vi "Main.vi"() -> ()   [LabVIEW 2013] (continued)
      n78 = control-ref of="Item Details"() -> (w112:refnum<vi>)
      n79 = control-ref of="WPS Details Setup"() -> (w111:refnum<vi>)
      n80 = control-ref of="Info. (Execute Page)"() -> (w96:refnum<vi>)
      n81 = control-ref of="Results Output"() -> (w72:refnum<vi>)
      n82 = control-ref of="Furnace Details"() -> (w98:refnum<vi>)
      n83 = control-ref of="Extra WPS"() -> (w110:refnum<vi>)
      n84 = control-ref of="Extra Rev"() -> (w109:refnum<vi>)
      n85 = control-ref of="Notes"() -> (w107:refnum<vi>)
      n86 = Initialize Array("", w121) -> (w242:string[])
      n87 = control-ref of="This Application"() -> (w187:refnum<vi>)
      n88 = Initialize Array("", w228) -> (w231:string[])
      n89 = Initialize Array("", w134) -> (w240:string[])
      n90 = property on="Tab Body" class="TabCtl (strict)" props=["Pages"]() -> ()  [unwired: 2 in, 3 out]
      n91 = property on="Tab Setup" class="TabCtl (strict)" props=["Pages"]() -> ()  [unwired: 2 in, 3 out]
      n92 = property on="Master Data Tab" class="TabCtl (strict)" props=["Pages"]() -> ()  [unwired: 2 in, 3 out]
      n93 = property class="App"(reference=w187) -> (error out=w142:errorcluster, "App.Dir"=w149:path, "App.Name"=w148:string)  [unwired: 1 in, 1 out]
      "Application:Name" <- w148
      "LabVIEW Directory Path" <- w149
      n94 = Build Array(w242) -> (w243:string[][])
      n95 = Build Array(w231) -> (w230:string[][])
      n96 = Build Array(w240) -> (w133:string[][])
      n97 = control-ref of="Equipment Details"() -> (w157:refnum<vi>)
      n98 = control-ref of="FTP File List"() -> (w126:refnum<vi>)
      n99 = control-ref of="Report List"() -> (w153:refnum<vi>)
      n100 = control-ref of="Part Details"() -> (w233:refnum<vi>)
      n101 = property on="MCListBox FHS Setup" class="MCListbox (strict)"("ItemNames"=w230, "NumCols"=w228, "ColHdrString"=w199) -> ()  [unwired: 2 in, 2 out]
      n102 = property on="MCListBox FHS Master Data" class="MCListbox (strict)"("ItemNames"=w243, "NumCols"=w121, "ColHdrString"=w199) -> ()  [unwired: 2 in, 2 out]
      n103 = property on="MCListBox AWPS" class="MCListbox (strict)"("ItemNames"=w133, "NumCols"=w134) -> ()  [unwired: 2 in, 2 out]
      n104 = Bundle By Name(cluster=T23 {"Item Details"=refnum, "WPS Details"=refnum, "WPS (Extra)"=refnum, "Rev (Extra) "=refnum, "FHS MCListbox"=refnum, "Additional WPS/Ref MCListBox"=refnum, "Notes"=refnum, "Part Details (MClistBox)"=refnum, "Result Output"=refnum} ("Refnums"), "Item Details"=w112, "WPS Details"=w111, "WPS (Extra)"=w110, "Rev (Extra)"=w109, "FHS MCListbox"=w114, "Additional WPS/Ref MCListBox"=w108, "Notes"=w107, "Part Details (MClistBox)"=w106, "Result Output"=w72) -> (→"DB Refnums":T23)
      n105 = Bundle By Name(cluster=T24 {"Furnace Details"=refnum, "CompactRIO Module Details"=refnum, "Info. (Execute Tab)"=refnum} ("DB Refnums II"), "Furnace Details"=w98, "CompactRIO Module Details"=w97, "Info. (Execute Tab)"=w96) -> (→"DB Refnums II":T24)
      n106 = control-ref of="MCListBox FHS Setup"() -> (w118:refnum<vi>)
      n107 = control-ref of="MCListBox FHS Master Data"() -> (w120:refnum<vi>)
      n108 = control-ref of="MCListBox AWPS"() -> (w179:refnum<vi>)
      n109 = property on="Material Copy" class="Bool"("DisabledEnum"=T30."Disabled and Grayed Out" ("Disabled")) -> ()  [unwired: 2 in, 2 out]
      n110 = property on="Material Paste" class="Bool"("DisabledEnum"=T30."Disabled and Grayed Out" ("Disabled")) -> ()  [unwired: 2 in, 2 out]
      n111 = Build Path(base path=w149, name or relative path=w148) -> (appended path=w147:path)
      n112 = Path To String(path=w147) -> (string=w146:string)
      n113 = invoke class="FileVersionInfo" method="GetVersionInfo"(error in=w142, "fileName"=w146) -> (reference out=w143:refnum<k24>, error out=w141:errorcluster, "GetVersionInfo"=w145:refnum<k24>)  [unwired: 2 in, 1 out]
      n114 = property class="MCListbox (strict)"(reference=w233, "ColHdrString"=w232, "NumRows"=w135, "NumCols"=u32 19 ("Number of Rows")) -> (reference out=w136:refnum<vi>)  [unwired: 1 in, 1 out]
      n115 = for {
        N: w135 -> [_]
        tunnel: w136 -> [w302]
        i -> [w301]
        n116 = for {
          N: 6 -> [_]
          tunnel: w302 -> [w309]
          tunnel: w301 -> [w306]
          tunnel: 13 -> [w305]
          i -> [w304]
          n117 = Add(x=w305, y=w304) -> (x+y=w303:i32)
          n118 = Bundle(w306, w303) -> (w307:cluster{i32, i32})  [unwired: 1 in]
          n119 = property class="MCListbox (strict)"(reference=w309, "ActiveCell"=w307, "Justify"=enum16{"Left", "Center", "Right"}."Center" ("Active Cell:Cell Justification")) -> ()  [unwired: 1 in, 2 out]
        }
      }
      n120 = property class="MCListbox (strict)"(reference=w157, "ColHdrString"=w154, "NumRows"=u32 4 ("Number of Rows"), "NumCols"=u32 5 ("Number of Rows")) -> (reference out=w156:refnum<vi>)  [unwired: 1 in, 1 out]
      n121 = property class="MCListbox (strict)"(reference=w153, "ColHdrString"=w150, "NumRows"=u32 5 ("Number of Rows"), "NumCols"=u32 7 ("Number of Rows")) -> (reference out=w152:refnum<vi>)  [unwired: 1 in, 1 out]
      n122 = property class="MCListbox (strict)"(reference=w126, "ColHdrString"=string[] ["Date and Time", "Transaction No."] ("Column Header Strings[]"), "NumRows"=u32 5 ("Number of Rows"), "NumCols"=u32 2 ("Number of Rows")) -> (reference out=w123:refnum<vi>)  [unwired: 1 in, 1 out]
      n123 = property on="Property Node" class="MCListbox (strict)"(reference=w120, "NumRows"=8 ("Multicolumn Listbox"), "TopLeft"=w173) -> ()  [unwired: 1 in, 2 out]
      n124 = property on="Property Node" class="MCListbox (strict)"(reference=w118, "NumRows"=8 ("Multicolumn Listbox"), "TopLeft"=w173) -> ()  [unwired: 1 in, 2 out]
      n125 = local write "Close"(FALSE ("Quit")) -> ()
      n126 = Build Array(w118, w120, w179) -> (w190:refnum<vi>[])
      "MCListBox Ref" <- w190
      n127 = property on="Part Details Add" class="Bool (strict)"("BoolText.Text"="Add" ("Boolean Text.Text"), "DisabledEnum"=T30."Enabled" ("Disabled")) -> ()  [unwired: 2 in, 2 out]
      n128 = property class="FileVersionInfo"(reference=w145, error in=w141) -> (reference out=w144:refnum<k24>, error out=w140:errorcluster, "FileVersion"=w137:string)
      n129 = for {
        tunnel: w190 -> [w362] mode=indexing
        tunnel: "CellBG Unused Cells" -> [w365]
        tunnel: "CellBG ColHdrs" -> [w364]
        tunnel: "CellBG New Cells" -> [_]
        n130 = property on="Property Node" class="MCListbox (strict)"(reference=w362, "RowHdrs[]"=string[] ["-1,-1", "", "0,0", "-1,-1", "7"]) -> (reference out=w361:refnum<vi>)  [unwired: 1 in, 1 out]
        n131 = property on="Property Node" class="MCListbox (strict)"(reference=w361, "ActiveCell"=T33 {"Row"=-2, "Column"=-2}, "CellBG"=w365, "ActiveCell"=T33 {"Row"=-1, "Column"=-2}, "CellBG"=w364, "Value"=-1 ("Multicolumn Listbox")) -> ()  [unwired: 1 in, 2 out]
      }
      n132 = Concatenate Strings("ver. ", w137) -> (w51:string)
      "File Version" <- w51
      n133 = flat-sequence "RSS Copyright" {
        frame #0 {
          # "Copyright (c) 2014, Reinehold Systems Solutions Pte Ltd. All Rights Reserved.\n\nThis application code (VI) is confidential and/or proprietary and is intended for the express use of the copyright owner and/or IP owner. This code is delivered as part of the Stress Relief Recording System. Any unauthorized re-use of this code outside of the Stress Relief Recording System is prohibited and punishable by law."
        }
      }
      n134 = flat-sequence "Report TAB" {
        frame #0 {
        }
      }
      n135 = Close Reference(reference=w144, error in (no error)=w140) -> (error out=w139:errorcluster)
      n136 = call "Get INFO from ini FILE - SRTRS.vi"("ini Name"="SRTRS.ini") -> ("Settings"=w56:T37, "Equipment Details (MCListBox)"=w214:string[][], "Furnace Details"=→"Furnace Details":T6, "SRTRS Connection Information"=w92:T38, "CMS Connection Information"=w80:T38, "AMS Connection Information"=w49:T38, "MessageQ"=w185:string, "Settings Boolean"=w48:T39, "Error Out"=w77:errorcluster)  [unwired: 5 in, 1 out]
      "ini File Error" <- w77
      n137 = Unbundle By Name(w56) -> ("cRIO IP"=w196:string, "Host COM Port"=w57:string, "Temperature Units"=w84:string, "cRIO Folder"=→"cRIO Folder":string, "cRIO Data Retention"=w177:string, "cRIO Time Sync Schedule"=w63:string, "cRIO Time Sync Tolerance"=w64:string, "Furnace Number"=→"Furnace Number":string, "Software Solution Name"=→"ApplicationName":string, "LogoFile"=w90:string, "Channel to Probe Mapping"=w211:string, "Running Number"=w213:string, "Permitted Temperature Difference"=w201:string, "Host Sampling Interval"=w189:string, "Latest stp File"=w131:string, "Log Off Timer"=w91:string, "Raw Data File"=→"Raw Data File":string, "SRTRS4070 Host Folder"=w36:string, "SRTRS4070 Folder"=→"SRTRS4070 Folder (Server Folder)":string, "Layout Details"=w34:string, "Date Format"=w26:string)  [unwired: 1 out]
      "cRIO IP" <- w196
      "Host COM Port" <- w57
      "SRTRS4070 Host Folder" <- w36
      n138 = Close Reference(reference=w143, error in (no error)=w139) -> ()  [unwired: 1 out]
      n139 = Build Array(w136, w156, w152, w123) -> (w244:refnum<vi>[])
      n140 = local read "CellBG Unused Cells"() -> (w234:u32)
      n141 = Concatenate Strings("{Initialization} SRTRS Initialize OK." ("string"), w185, " " ("string"), w181) -> (w28:string)
      n142 = Unbundle By Name "Settings Boolean"(w48) -> ("Create EXCEL"=w205:bool, "Create PDF"=w204:bool, "Use Host COM Port"=w195:bool, "Show LabVIEW Error"=→"Show LabVIEW Error":bool, "Show Debug Tab"=w39:bool, "Show Scrollbars"=w163:bool, "Stop On Final Target Temperature"=w129:bool, "Update English Captions"=w40:bool)
      "Show Debug TAB" <- w39
      "Show Scrollbars" <- w163
      "Update English Captions" <- w40
      n143 = Select(t=T31."Always On" ("Vertical Scrollbar Visibility"), s=w163, f=T31."Off While Running" ("Vertical Scrollbar Visibility")) -> (s? t:f=w160:T31)
      n144 = property class="Pane"(reference=w164, "HorizScrollbarVisibility"=w160, "VertScrollbarVisibility"=w160) -> ()  [unwired: 1 in, 2 out]
      n145 = Unbundle By Name "Settings Boolean"(w48) -> ("Simulate cRIO"=w47:bool, "Simulate ET3500"=w46:bool, "Simulate No DB"=w44:bool, "Lite Version"=w45:bool)
      "Lite Version" <- w45
      n146 = case shown="True" "DB - Logon" {
        frame False {
        }
        frame True {
          n147 = property on="Close" class="Bool (strict)"("BoolText.Text"="Log off" ("Label.Text")) -> (error out=w276:errorcluster)  [unwired: 2 in, 1 out]
          n148 = property on="Close" class="Bool (strict)"(error in=w276, "Val(Sgnl)"=TRUE ("Value (Signaling)")) -> ()  [unwired: 1 in, 2 out]
        }
      }
      n149 = for {
        tunnel: w244 -> [w371] mode=indexing
        tunnel: w234 -> [w370]
        tunnel: string[][] [] ("Item Names") -> [w369]
        w372 = T33 {"Row"=-1, "Column"=-2}  # All ColHdrs
        w373 = T33 {"Row"=-2, "Column"=-2}  # All Rows & Columns (Including Headers)
        n150 = property on="Property Node" class="MCListbox (strict)"(reference=w371, "ActiveCell"=w373, "CellBG"=w370, "ActiveCell"=w372, "CellBG"=u32 12105912, "ItemNames"=w369) -> ()  [unwired: 1 in, 2 out]
      }
      n151 = Reverse String(1:w51) -> (0:w52:string)
      n152 = local write "Date Format (UserDefined)"(w26) -> ()
      n153 = Match Pattern(string=w52, regular expression="\\." ("search string")) -> (after substring=w54:string)  [unwired: 1 in, 3 out]
      n154 = flat-sequence "MasterData TAB (xx Controls)" {
        frame #0 {
          n155 = property on="SAPMaterial Description (Long) Master Data Tab" class="Bool"("DisabledEnum"=T30."Disabled and Grayed Out" ("Disabled")) -> ()  [unwired: 2 in, 2 out]
          n156 = property on="Master Data Material Description" class="Str"("Text.BGColor"=u32 16777215, "DisabledEnum"=T30."Enabled" ("Disabled")) -> ()  [unwired: 2 in, 2 out]
          n157 = property on="Material Save" class="Bool"("DisabledEnum"=T30."Disabled and Grayed Out" ("Disabled")) -> ()  [unwired: 2 in, 2 out]
        }
      }
      n158 = Search and Replace String(input string="ni.var.psp://cRIO IP/RT Library" ("String"), search string="cRIO IP" ("String"), replace string=w196) -> (result string=→"cRIO shared variable RT Library":string)  [unwired: 5 in, 3 out]
      n159 = Search and Replace String(input string="visa://cRIO IP/ASRL1::INSTR" ("String"), search string="cRIO IP" ("String"), replace string=w196) -> (result string=w194:string)  [unwired: 5 in, 3 out]
      "cRIO COM Port" <- w194
      n160 = Reverse String(1:w54) -> (0:→"Plant and Furnace Name" →"Plant and Furnace Name (B4 Logon)":string)
      n161 = local write "Use Host COM Port"(w195) -> ()
      n162 = local write "Report.Create.Excel"(w205) -> ()
      n163 = local write "Report.Create.PDF"(w204) -> ()
      n164 = global write "Global SRTRS.vi" "SRTRS Connection Information"(w92) -> ()
      n165 = global write "Global SRTRS.vi" "CMS Connection Information"(w80) -> ()
      n166 = global write "Global SRTRS.vi" "AMS Connection Information"(w49) -> ()
      n167 = property on="Equipment Details" class="MCListbox (strict)"("ItemNames"=w214) -> ()  [unwired: 2 in, 2 out]
      n168 = global write "Global SRTRS.vi" "Update English Captions"(w40) -> ()
      n169 = Decimal String To Number(string=w177) -> (number=→"cRIO Data Retention":i32)  [unwired: 2 in, 1 out]
      n170 = Decimal String To Number(string=w64) -> (number=→"cRIO Time Sync Tolerance":i32)  [unwired: 2 in, 1 out]
      n171 = Match Pattern(string=w63, regular expression=":") -> (before substring=w61:string, after substring=w60:string)  [unwired: 1 in, 2 out]
      n172 = String To Path(string=w131) -> (path=→"Latest stp file":path)
      n173 = Bundle("Channel to Probe Mapping"=w211) -> (w172:cluster{"Channel to Probe Mapping":string})  [unwired: 1 in]
      n174 = Decimal String To Number(string=w213) -> (number=→"Running Number":i32)  [unwired: 2 in, 1 out]
      n175 = String To Path(string=w90) -> (path=w89:path)
      n176 = Fract/Exp String To Number(string=w201) -> (number=w200:dbl)  [unwired: 3 in, 1 out]
      n177 = Fract/Exp String To Number(string=w189) -> (number=→"Host Sampling Interval (s)":dbl)  [unwired: 3 in, 1 out]
      n178 = Decimal String To Number(string=w91) -> (number=→"Log Off Timer (s)":i32)  [unwired: 2 in, 1 out]
      n179 = Match Pattern(string=w34, regular expression="\t" ("search string/char (-)")) -> (before substring=→"Layout ID":string, after substring=w32:string)  [unwired: 1 in, 2 out]
      n180 = property on="Channel to Probe Mapping" class="Clust (strict)"("Value"=w172) -> ()  [unwired: 2 in, 2 out]
      n181 = Concatenate Strings(w61, w60) -> (w59:string)
      n182 = property on="Variant Allowed (Hold Temp)" class="DigNum (strict)"("Value"=w200) -> ()  [unwired: 2 in, 2 out]
      n183 = call <vilib>:"Read JPEG File.vi"("path to JPEG file"=w89) -> ("error out"=→"LogoName":errorcluster, "image data"=w88:T40)  [unwired: 8 in, 1 out]
      n184 = String To Path(string=w32) -> (path=→"Template File":path)
      n185 = case shown="True" "Edit WPS in Setup" {
        tunnel: w120 -> [w280 w282]
        tunnel: [w281 w284] -> w119
        tunnel: w118 -> [_ w283]
        frame False {
          # "Only Master FHS"
          n186 = Build Array(w280) -> (w281:refnum<vi>[])
        }
        frame True {
          # "Both FHS"
          n187 = Build Array(w283, w282) -> (w284:refnum<vi>[])
        }
      }
      n188 = Decimal String To Number(string=w59) -> (number=→"cRIO Time Sync Schedule":i32)  [unwired: 2 in, 1 out]
      n189 = call <vilib>:"Draw Flattened Pixmap.vi"("image data"=w88) -> ("new picture"=→"LogoName":picture)  [unwired: 8 in]
      n190 = case shown="True" w45 {
        tunnel: w47 -> [w296 _]
        tunnel: [w296 w298] -> w128
        tunnel: w46 -> [w295 _]
        tunnel: [w295 w298] -> w127
        frame False {
          # "Set Focus on Setup Tab"
          # "Full Version"
          n191 = property on="Tab Setup" class="TabCtl (strict)"("Value"=enum32{"Part Details", "Furnace Settings"}."Part Details" ("Tab Setup")) -> ()  [unwired: 2 in, 2 out]
        }
        frame True {
          w298 = TRUE ("Simulate cRIO")
          # "Simulate cRIO and ET3500"
          # "Lite Version"
        }
      }
      n192 = case shown="False" w44 {
        tunnel: [i32[] [0, 1, 2] i32[] [1]] -> w43
        tunnel: [TRUE FALSE] -> w42
        frame False {
          # "2 - Caption"
          # "DB Availiable"
        }
        frame True {
          # "Skip 0"
          # "Simulate No DB"
        }
      }
      "Settings Load Sequence" <- w43
      n193 = local write "Stop On Final Target Temperature"(w129) -> ()
      n194 = local write "From Search Button"(FALSE ("From Search Button")) -> ()
      n195 = for {
        tunnel: "CellBG New Cells" -> [w289]
        tunnel: w119 -> [w286] mode=indexing
        # "MClistbox FHS Setup \nis set to FALSE for\n\"Allowing Editing Cells\"\n/\"Editable Cells"
        # "Create WHITE\neditable cells"
        n196 = property on="Property Node" class="MCListbox (strict)"(reference=w286, "Allow Editing Cells"=TRUE) -> (reference out=w288:refnum<vi>, "NumCols"=w287:u32)  [unwired: 1 in, 1 out]
        n197 = for {
          N: w287 -> [_]
          tunnel: w289 -> [w291]
          tunnel: w288 -> [w290]
          i -> [w293]
          n198 = Bundle("Multicolumn Listbox"=0, w293) -> (w292:cluster{"Multicolumn Listbox":i32, i32})  [unwired: 1 in]
          n199 = property on="Property Node" class="MCListbox (strict)"(reference=w290, "ActiveCell"=w292, "CellBG"=w291) -> ()  [unwired: 1 in, 2 out]
        }
      }
      n200 = control-ref of="Logs_Host"() -> (w38:refnum<vi>)
      n201 = flat-sequence "Admin TAB (xx Controls)" {
        frame #0 {
        }
      }
      n202 = control-ref of="Master Data Temperature Units"() -> (w227:refnum<vi>)
      n203 = control-ref of="Key Values Temperature Units"() -> (w226:refnum<vi>)
      n204 = control-ref of="WPS Details Temperature Units"() -> (w225:refnum<vi>)
      n205 = control-ref of="Info. Temperature Units"() -> (w223:refnum<vi>)
      n206 = control-ref of="Info. Temperature Units 2"() -> (w222:refnum<vi>)
      n207 = control-ref of="FHS Ramp Rate Units"() -> (w209:refnum<vi>)
      n208 = control-ref of="FHS Target Temp Units"() -> (w208:refnum<vi>)
      n209 = control-ref of="MasterData FHS Ramp Rate Temp Units"() -> (w207:refnum<vi>)
      n210 = control-ref of="MasterData FHS Target Temp Units"() -> (w206:refnum<vi>)
      n211 = Select(t=w57, s=w195, f=w194) -> (s? t:f=→"VISA resource name RS232":string)
      n212 = local write "Extra WPS"(w122) -> ()
      n213 = local write "Extra Rev"(w122) -> ()
      n214 = Build Array(w38) -> (w37:refnum<vi>[])
      n215 = call "Folder - Create Application Folders.vi"("ControlsOnPage"=w37, "SRTRS4070 Folder"=w36) -> ("error out"=w35:errorcluster)  [unwired: 8 in, 1 out]
      n216 = property on="Setup Load Debug" class="Bool"("Visible"=w39) -> ()  [unwired: 2 in, 2 out]
      n217 = property on="[Remarks] +[ShortDescription] Debug" class="Str"("Visible"=w39) -> ()  [unwired: 2 in, 2 out]
      n218 = local write "Event File Error"(w35) -> ()
      n219 = Concatenate Strings("Temperature " ("string"), w84) -> (w158:string)
      n220 = Build Array(w227, w226, w225, w223, w222, w209, w208, w207, w206) -> (w224:refnum<vi>[])
      "Temperature Units" <- w224
      n221 = flat-sequence "Config TAB (xx Controls)" {
        frame #0 {
        }
      }
      n222 = property on="Chart" class="WFChart (strict)"("YScale.NameLbl.Text"=w158) -> ()  [unwired: 2 in, 2 out]
      n223 = local write "Simulate cRIO"(w128) -> ()
      n224 = local write "Simulate ET3500"(w127) -> ()
      n225 = for {
        tunnel: w224 -> [w356] mode=indexing
        tunnel: w84 -> [w355]
        n226 = property class="Str"(reference=w356, "Value"=w355) -> ()  [unwired: 1 in, 2 out]
      }
      n227 = global write "Global SRTRS.vi" "Temperature Units"(w84) -> ()
      n228 = Obtain Queue(max queue size (-1, unlimited)=10, name (unnamed)="MessageQ", element data type="", error in (no error)=w77) -> (queue out=w74:refnum<queue>, error out=w246:errorcluster)  [unwired: 1 in, 1 out]
      n229 = local write "DB - Master Data Save"(w42) -> ()
      n230 = local write "DB - Master Data Load"(w42) -> ()
      n231 = local write "DB - Setup Item (Part Details)"(w42) -> ()
      n232 = local write "DB - Transaction"(w42) -> ()
      n233 = local write "DB - Active Process"(w42) -> ()
      n234 = local write "DB - Report"(w42) -> ()
      n235 = local write "DB - Message"(w42) -> ()
      n236 = local write "DB - Logon"(TRUE ("DB - Logon")) -> ()
      n237 = flat-sequence "DEBUG TAB (xx Controls)" {
        frame #0 {
          n238 = property on="Paste Setup" class="Bool"("DisabledEnum"=T30."Disabled and Grayed Out" ("Disabled")) -> ()  [unwired: 2 in, 2 out]
          n239 = property on="Copy Setup" class="Bool"("DisabledEnum"=T30."Enabled" ("Disabled")) -> ()  [unwired: 2 in, 2 out]
        }
      }
      n240 = disable-structure shown="Enabled" {
        disable-tunnel: w246 -> [w265 w266]
        disable-tunnel: [w264 w266] -> w245
        disable-tunnel: w74 -> [w263 w267]
        disable-tunnel: [w262 w267] -> w73
        frame Disabled {
          n241 = Enqueue Element(queue=w263, error in (no error)=w265) -> (queue out=w262:refnum<queue>, error out=w264:errorcluster)  [unwired: 2 in, 1 out]
        }
        frame Enabled {
        }
      }
      n242 = call "Queue - EnQueue to MessageQ.vi"("<NoD> Don't Display to UI"=TRUE, "Message"=w28) -> ("Error Out"=w27:errorcluster)  [unwired: 9 in]
      n243 = global write "Global SRTRS.vi" "MessageQ"(w74) -> ()
      n244 = local write "MessageQ Error"(w27) -> ()
      "Recipe Start Flag" <- FALSE ("Recipe Start Flag")
      "Recipe Stop Flag" <- FALSE ("Recipe Stop Flag")
      "Quit Flag" <- FALSE ("Quit Flag")
      "Uploaded to ET" <- FALSE ("Quit Flag")
      "RecoveryFlag" <- FALSE ("RecoveryFlag")
      "Logon OK" <- FALSE ("Logon OK")
    }
  }
  n245 = Initialize Array("", w22) -> (w21:string[])
  n246 = while {
    tunnel: w20 -> [w385]
    shift-right: [w404] -> _
    shift-left: w21 -> [w406]
    shift-right: [w393] -> w19
    shift-left: _ -> [w392]
    shift-right: [w391] -> w18
    shift-left: _ -> [w390]
    tunnel: w2 -> [w386]
    tunnel: [w383] -> w6
    i -> [w396]
    stop <- w381 stop-if-true
    # "Need to take care of Unicode here"
    # "Event Structure For MessageQ"
    n247 = Dequeue Element(queue=w385, error in (no error)=w386) -> (element=w382:string, error out=w384:errorcluster)  [unwired: 1 in, 2 out]
    n248 = flat-sequence {
      tunnel: w396 -> [w477]
      tunnel: [w472] -> w403
      tunnel: w384 -> [w471]
      tunnel: [w471] -> w398
      tunnel: [w470] -> w380
      frame #0 {
        # "SERIAL No + Time Stamp"
        n249 = Format Date/Time String(time format string (%c)="%Y%m%d_%H%M%S") -> (date/time string=w470:string)  [unwired: 2 in]
        n250 = Format Into String(format string="%06d", w477) -> (resulting string=w474:string)  [unwired: 2 in, 1 out]
        n251 = Concatenate Strings(w474, "\t", w470) -> (w472:string)
      }
    }
    n252 = case shown="0" w396 {
      tunnel: w380 -> [w450 _]
      tunnel: [w441 w462] -> w395
      tunnel: [w447 w461] -> w394
      tunnel: w392 -> [_ w462]
      tunnel: w390 -> [_ w461]
      tunnel: w385 -> [w434 _]
      frame 0 {
        w438 = "\"" ("string")
        # "SRTRS4070 Host"
        # "Create .log Event File for 1st and only time"
        n253 = local read "Logs_Host"() -> (w430:path)
        n254 = Format Date/Time String(time format string (%c)="%Y\\%m") -> (date/time string=w433:string)  [unwired: 2 in]
        n255 = Build Path(base path=w430, name or relative path=w433) -> (appended path=w431:path)
        n256 = call <vilib>:"Check if File or Folder Exists.vi"("path"=w431) -> ("error out"=w444:errorcluster, "file or folder exists?"=w446:bool, "dup path"=w445:path)  [unwired: 8 in]
        n257 = case shown="False" w446 {
          tunnel: w445 -> [w458 w460]
          tunnel: [w457 w460] -> w443
          tunnel: [w456 w459] -> w442
          tunnel: w444 -> [w455 w459]
          frame False {
            # "Create Folder if NOT found\nCreate NEW"
            n258 = Create Folder(path (use dialog)=w458, error in=w455) -> (created path=w457:path, error out=w456:errorcluster)  [unwired: 1 in, 1 out]
          }
          frame True {
            # "Folder Found"
          }
        }
        n259 = Concatenate Strings(w450, ".log" ("string")) -> (w448:string)
        n260 = Build Path(base path=w443, name or relative path=w448) -> (appended path=w437:path)
        n261 = Open/Create/Replace File(file path (use dialog)=w437, error in=w442, operation (0:open)=T41."replace or create", access (0:read/write)=enum16{"read/write", "read-only", "write-only"}."write-only") -> (refnum out=w441:refnum<file>, error out=w447:errorcluster)  [unwired: 2 in, 1 out]
        n262 = Not A Number/Path/Refnum?(number/path/refnum=w441) -> (NaN/Path/Refnum?=w440:bool)
        n263 = case shown="False" w440 {
          tunnel: [" Event File Created. <NoD>" ("string") " Event File Not Created. <NoD>" ("string")] -> w436
          frame False {
            # "File Load OK"
          }
          frame True {
            # "File Not Loaded"
          }
        }
        n264 = Path To String(path=w437) -> (string=w439:string)
        n265 = Concatenate Strings(w438, w439, w438, w436) -> (w435:string)
        n266 = Enqueue Element(queue=w434, element=w435) -> ()  [unwired: 2 in, 3 out]
      }
      frame 1, Default {
      }
    }
    n267 = disable-structure shown="Enabled" {
      disable-tunnel: w382 -> [w413 w416]
      disable-tunnel: [w412 w416] -> w379
      frame Disabled {
        # "Remove all \\n Replace with space\nFor display in .Log file"
        n268 = call <vilib>:"Space Constant.vi"() -> ("String"=w411:string)
        n269 = call <vilib>:"Search and Replace Pattern.vi"("string"=w413, "regular expression (\"\")"="\n", "replace string (\"\")"=w411, "replace all? (F)"=TRUE) -> ("result string"=w412:string)  [unwired: 1 in, 1 out]
      }
      frame Enabled {
      }
    }
    n270 = case shown="No Error" w398 {
      selector: w398 -> [w463 w464]
      tunnel: [_ w465] -> w401
      tunnel: [w463 w464] -> w383
      frame No Error {
      }
      frame Error {
        n271 = Unbundle By Name(w464) -> ("source"=w469:string)
        n272 = Concatenate Strings("\t" ("string"), "[ERROR " ("format string"), w469, "]" ("string")) -> (w465:string)
      }
    }
    n273 = Rotate 1D Array(1:w406, 2:1 ("n")) -> (0:w409:string[])
    n274 = Match Pattern "QUIT is ISSUED"(string=w379, regular expression="QUIT") -> (offset past match=w399:i32)  [unwired: 1 in, 3 out]
    n275 = Concatenate Strings(w403, "\t" ("string"), w379, w401) -> (w389:string)
    n276 = Greater Or Equal To 0?(x=w399) -> (x >= 0?=w397:bool)
    n277 = Replace Array Subset(array=w409, new element=w389) -> (w404:string[])  [unwired: 1 in]
    n278 = Concatenate Strings(w389, "\n" ("delimiter (Tab)")) -> (w387:string)
    n279 = Write to Text File(file (use dialog)=w395, text=w387, error in=w394) -> (refnum out=w393:refnum<file>, error out=w391:errorcluster)  [unwired: 1 in, 1 out]
    n280 = Or(x=w383, y=w397) -> (x .or. y?=w381:bool)
    n281 = Search and Replace String(replace all?=FALSE ("replace all? (F)"), input string=w379, search string="<NoD>") -> (result string=w375:string, number of replacements=w377:i32)  [unwired: 5 in, 2 out]
    n282 = Array To Spreadsheet String(delimiter (Tab)="\n", array=w404, 3:"" ("format string")) -> (spreadsheet string=→"MessageQ":string)
    n283 = Greater Than 0?(x=w377) -> (x > 0?=w376:bool)
    n284 = case shown="False" w376 {
      tunnel: w375 -> [w422 _]
      frame False {
        # "/* These are hidden    */"
        # "Display"
        n285 = disable-structure shown="Enabled" {
          disable-tunnel: w422 -> [w427 w429]
          disable-tunnel: [w426 w429] -> w419
          frame Disabled {
            n286 = global read "Global SRTRS.vi" "Date Time Format"() -> (w428:string)
            n287 = Format Date/Time String(time format string (%c)=w428) -> (date/time string=w425:string)  [unwired: 2 in]
            n288 = call-poly "Tool_Unicode Convert ASCII to Unicode.vi"("ASCII"=w425) -> ("Unicode"=w424:string)  [unwired: 4 in]
            n289 = Concatenate Strings(w424, " \u0000" ("string"), w427) -> (w426:string)
          }
          frame Enabled {
          }
        }
        n290 = Match Pattern(string=w419, regular expression="//*.*/*/") -> (before substring=w420:string, after substring=w418:string)  [unwired: 1 in, 2 out]
        n291 = Concatenate Strings(w420, w418) -> (→"[Remarks] +[ShortDescription]" →"[Remarks] +[ShortDescription] Debug":string)
      }
      frame True {
        # "Do Not Display"
      }
    }
  }
  "MessageQ Error" <- w6
  n292 = while {
    tunnel: [w492] -> _
    tunnel: w20 -> [_]
    shift-right: [w490] -> _
    shift-left: FALSE -> [w491]
    shift-right: [w479] -> w4
    shift-left: _ -> [w478]
    stop <- w492 stop-if-true
    # "Event Structure For UIEvents                                                                      Event Structure For UIEvents                                                                   Event Structure For UIEvents                                                                       Event Structure For UIEvents                                                                                      Event Structure For UIEvents"
    n293 = control-ref of="Part Details"() -> (w482:refnum<vi>)
    n294 = control-ref of="MCListBox FHS Setup"() -> (w489:refnum<vi>)
    n295 = control-ref of="MCListBox AWPS"() -> (w488:refnum<vi>)
    n296 = control-ref of="Equipment Details"() -> (w487:refnum<vi>)
    n297 = control-ref of="WPS Details Setup"() -> (w484:refnum<vi>)
    n298 = control-ref of="Additional WPS/Ref"() -> ()  [unwired: 1 out]
    n299 = control-ref of="Furnace Details"() -> (w485:refnum<vi>)
    n300 = control-ref of="Channel to Probe Mapping"() -> (w481:refnum<vi>)
    n301 = local read "MCListBox Ref"() -> (w480:refnum<vi>[])
    n302 = Build Array "Part Details \nMCListbox"(w482, w489, w488, w487) -> (w486:refnum<vi>[])
    n303 = Build Array "Part Details\nClusters"(w484, w485, w481) -> (w483:refnum<vi>[])
    n304 = event shown="[38] \"Report Generate Toggle\": Value Change" {
      selector: _ -> [_ _ _ _ _ _ _ _ _ _ _ _ _ _ _ _ _ _ _ _ _ _ _ _ _ _ _ _ _ _ _ _ _ _ _ _ _ _ _ _ _ _ _ _ _ _ _ _ _ _ _ _ _ _ _ _ _ _ _ _ _ _ _ _ _ _ _ _ _ _ _ _ _ _ _ _ _ _ _ _ _ _ _ _]
      dyn-events: _ -> [_ _ _ _ _ _ _ _ _ _ _ _ _ _ _ _ _ _ _ _ _ _ _ _ _ _ _ _ _ _ _ _ _ _ _ _ _ _ _ _ _ _ _ _ _ _ _ _ _ _ _ _ _ _ _ _ _ _ _ _ _ _ _ _ _ _ _ _ _ _ _ _ _ _ _ _ _ _ _ _ _ _ _ _]
      timeout: _ -> [_ _ _ _ _ _ _ _ _ _ _ _ _ _ _ _ _ _ _ _ _ _ _ _ _ _ _ _ _ _ _ _ _ _ _ _ _ _ _ _ _ _ _ _ _ _ _ _ _ _ _ _ _ _ _ _ _ _ _ _ _ _ _ _ _ _ _ _ _ _ _ _ _ _ _ _ _ _ _ _ _ _ _ _]
      tunnel: [_ _ _ _ w638 _ _ _ _ _ _ _ _ _ _ _ _ _ _ _ _ _ _ _ _ _ _ _ _ _ _ _ _ _ _ _ _ _ _ _ _ _ _ _ _ _ _ _ _ _ _ _ _ _ _ _ _ _ _ _ _ _ _ _ _ _ _ _ _ _ _ _ _ _ _ _ _ _ _ _ _ _ _ _] -> w492
      tunnel: w491 -> [_ _ _ _ _ _ _ _ _ _ _ _ _ _ _ _ _ _ _ _ _ _ _ _ _ _ _ _ _ _ _ _ _ _ _ _ _ _ _ _ _ _ _ _ _ w2772 _ _ _ _ _ _ _ _ _ _ _ _ _ _ _ _ _ _ _ _ _ _ _ _ _ _ _ _ _ _ _ _ _ _ _ _ _ _]
      tunnel: [_ _ _ _ _ _ _ _ _ _ _ _ _ _ _ _ _ _ _ _ _ _ _ _ _ _ _ _ _ _ _ _ _ _ _ _ _ _ _ _ _ _ _ _ _ TRUE _ _ _ _ _ _ _ _ _ _ _ _ _ _ _ _ _ _ _ _ _ _ _ _ _ _ _ _ _ _ _ _ _ _ _ _ _ _] -> w490
      tunnel: w486 -> [_ _ _ _ _ _ _ _ w840 _ _ _ _ _ _ _ _ _ _ _ _ w1463 _ w1512 _ _ _ _ _ _ _ _ _ _ _ _ _ _ w2213 _ _ _ _ _ _ _ _ _ _ _ _ _ _ _ _ _ _ _ _ _ _ _ _ _ _ _ _ _ _ _ _ _ _ _ _ _ _ _ _ _ _ _ _ _]
      tunnel: w483 -> [_ _ _ _ _ _ _ _ w846 _ _ _ _ _ _ _ _ _ _ _ _ _ _ _ _ _ _ _ _ _ _ _ _ _ _ _ _ _ w2212 _ _ _ _ _ _ _ _ _ _ _ _ _ _ _ _ _ _ _ _ _ _ _ _ _ _ _ _ _ _ _ _ _ _ _ _ _ _ _ _ _ _ _ _ _]
      tunnel: w482 -> [_ _ _ _ _ _ _ _ _ _ _ _ _ _ _ _ _ _ _ _ _ _ _ _ _ _ _ _ _ _ _ _ _ _ _ _ _ _ _ _ _ _ _ _ _ _ _ _ _ _ _ w3188 _ _ _ _ _ _ _ w3336 _ _ _ _ _ _ _ _ _ _ _ _ _ _ _ _ _ _ _ _ _ _ _ _]
      tunnel: w480 -> [_ _ _ _ _ _ _ _ _ _ _ _ _ _ _ _ _ _ _ _ _ _ _ _ _ _ _ _ _ _ _ _ _ _ _ _ _ _ _ _ _ _ _ _ w2731 _ _ _ _ _ _ _ _ _ _ _ _ _ _ _ _ _ _ _ _ _ _ _ _ _ _ _ _ _ _ _ _ _ _ _ _ _ _ _]
      tunnel: [_ w497 _ _ _ _ _ _ _ _ _ _ _ _ _ _ _ _ _ _ _ _ _ _ _ _ _ _ _ _ _ _ _ _ _ _ _ _ _ _ _ _ _ _ _ _ _ _ _ _ _ _ _ _ _ _ _ _ _ _ _ _ _ _ _ _ _ _ _ _ _ _ _ _ _ _ _ _ _ _ _ _ _ _] -> w479
      tunnel: w478 -> [_ w496 _ _ _ _ _ _ _ _ _ _ _ _ _ _ _ _ _ _ _ _ _ _ _ _ _ _ _ _ _ _ _ _ _ _ _ _ _ _ _ _ _ _ _ _ _ _ _ _ _ _ _ _ _ _ _ _ _ _ _ _ _ _ _ _ _ _ _ _ _ _ _ _ _ _ _ _ _ _ _ _ _ _]
      event Timeout {
        n305 = event-data() -> ()  [unwired: 1 in, 3 out]
      }
      event "Tab Body": Value Change {
        w493 = ""
        # "Clears When TAB is changed"
        n306 = event-data() -> ("NewVal"=w495:T1)  [unwired: 1 in, 5 out]
        n307 = case shown="\"Setup\", Default" w495 {
          selector: w495 -> [w498 w500]
          tunnel: [w498 w501] -> w494
          frame "Setup", Default {
          }
          frame "Master Data" {
            w499 = T1."Setup"  # Do Nothing
            n308 = property on="Master Data Tab" class="TabCtl (strict)"() -> ("Value"=w504:enum32{"Material", "WPS", "Layout"})  [unwired: 2 in, 2 out]
            n309 = Equal?(x=w504, y=enum32{"Material", "WPS", "Layout"}."Layout") -> (x = y?=w502:bool)
            n310 = Select(t=w500, s=w502, f=w499) -> (s? t:f=w501:T1)
          }
        }
        n311 = local write "[Remarks] +[ShortDescription] Debug"(w493) -> ()
        n312 = local write "[Remarks] +[ShortDescription]"(w493) -> ()
        n313 = case shown="\"Master Data\"..\"Logon\"" w494 {
          selector: w494 -> [_ w509 _]
          tunnel: [w505 w525 w611] -> w497
          tunnel: w496 -> [w505 _ w611]
          frame "Setup", "Debug", Default {
            # "Default Event. Do Nothing here."
          }
          frame "Master Data".."Logon" {
            # "SubPanel VI's Path\n..\\SRTRS\\VIs\\SubPanels\\DB UI - Logon.vi\nOR \n..\\SRTRS\\SRTRS.exe\\SubPanels\\DB UI - Logon.vi"
            # "Current VI's Path\n..\\SRTRS\\VIs\\Main.vi\nOR \n..\\SRTRS\\SRTRS.exe\\Main.vi"
            # "C:\\Users\\CK\\workspace\\LabVIEW\\Stress Relief Temperature Recording\\VIs\\SubPanels\\DB - Config UI.vi"
            # "Master Data, Admin, Config, Logon"
            n314 = case shown="\"Config\", Default" w509 {
              tunnel: ["DB UI - Config.vi" ("name or relative path") w541 "DB UI - Logon.vi" ("name or relative path") w549] -> w508
              tunnel: [w537 w540 w545 w548] -> w518
              frame "Config", Default {
                # "Config"
                n315 = control-ref of="Config UI"() -> (w537:refnum<vi>)
              }
              frame "Master Data" {
                # "Master Data CHILD TAB"
                n316 = property on="Master Data Tab" class="TabCtl (strict)"() -> ("Value"=w539:enum32{"Material", "WPS", "Layout"})  [unwired: 2 in, 2 out]
                n317 = case shown="\"Layout\"" w539 {
                  tunnel: [_ "DB UI - Master Data Layout.vi" ("name or relative path")] -> w541
                  tunnel: [_ w542] -> w540
                  frame Default {
                  }
                  frame "Layout" {
                    n318 = control-ref of="Layout UI"() -> (w542:refnum<vi>)
                  }
                }
              }
              frame "Logon" {
                n319 = control-ref of="Logon UI"() -> (w545:refnum<vi>)
                n320 = property on="Close" class="Bool (strict)"("BoolText.Text"="Close") -> ()  [unwired: 2 in, 2 out]
              }
              frame "Admin" {
                # "User or Equipment CHILD TAB"
                n321 = property on="Admin (User/Equipment) Tab" class="TabCtl (strict)"() -> ("Value"=w547:enum32{"User", "Equipment"})  [unwired: 2 in, 2 out]
                n322 = case shown="\"User\", Default" w547 {
                  tunnel: ["DB UI - Admin User.vi" ("name or relative path") "DB UI - Admin Equipment.vi" ("name or relative path")] -> w549
                  tunnel: [w551 w552] -> w548
                  frame "User", Default {
                    n323 = control-ref of="Admin User UI"() -> (w551:refnum<vi>)
                  }
                  frame "Equipment" {
                    n324 = control-ref of="Equipment UI"() -> (w552:refnum<vi>)
                  }
                }
              }
            }
            n325 = local read "Current VI's path"() -> (w513:path)
            n326 = Strip Path(path=w513) -> (stripped path=w510:path)  [unwired: 1 out]
            n327 = Build Path(base path=w510, name or relative path="SubPanels") -> (appended path=w512:path)
            n328 = Build Path(base path=w512, name or relative path=w508) -> (appended path=w524:path)
            n329 = Open VI Reference(vi path=w524, error in (no error)=errorcluster {"status"=FALSE, "code"=0, "source"=""} ("error constant")) -> (vi reference=w519:refnum<vi>, error out=w526:errorcluster)  [unwired: 4 in]
            n330 = property class="VI"(reference=w519) -> (reference out=w523:refnum<vi>, "Exec.State"=w521:T26, "FP.State"=→"Front Panel Window:State":T27)  [unwired: 1 in, 1 out]
            "Execution:State" <- w521
            n331 = case shown="\"Admin\"" w509 {
              tunnel: w519 -> [w528 w529 w531 w535]
              frame "Config", Default {
                # "Config"
                "Config UI" <- w528
              }
              frame "Logon" {
                "Logon UI" <- w529
              }
              frame "Admin" {
                # "User or Equipment CHILD TAB"
                n332 = property on="Admin (User/Equipment) Tab" class="TabCtl (strict)"() -> ("Value"=w530:enum32{"User", "Equipment"})  [unwired: 2 in, 2 out]
                n333 = case shown="\"Equipment\"" w530 {
                  tunnel: w531 -> [w532 w533]
                  frame "User", Default {
                    "Admin User UI" <- w532
                  }
                  frame "Equipment" {
                    "Admin Equipment UI" <- w533
                  }
                }
              }
              frame "Master Data" {
                # "User or Equipment CHILD TAB"
                n334 = property on="Master Data Tab" class="TabCtl (strict)"() -> ("Value"=w534:enum32{"Material", "WPS", "Layout"})  [unwired: 2 in, 2 out]
                n335 = case shown="\"Layout\"" w534 {
                  tunnel: w535 -> [_ w536]
                  frame Default {
                  }
                  frame "Layout" {
                    "Layout UI" <- w536
                  }
                }
              }
            }
            n336 = case shown="\"Idle\"" w521 {
              tunnel: w526 -> [w555 w585]
              tunnel: [w554 w583] -> w525
              tunnel: w523 -> [w556 w577]
              tunnel: ["UI Already Loaded" ("string") " UI Load OK." ("string")] -> w520
              tunnel: w518 -> [_ w575]
              tunnel: w509 -> [_ w569]
              tunnel: w508 -> [_ w566]
              frame "Running", Default {
                # "Close Each time to release the Ref.\nA new Ref will be created each time use Changes\nTab. No problem here because VI still Running."
                # "Already Running"
                n337 = Close Reference(reference=w556, error in (no error)=w555) -> (error out=w554:errorcluster)
              }
              frame "Idle" {
                w580 = T31."Off While Running" ("Horizontal Scrollbar Visibility")
                # "SubPanel VI's Path\n..\\SRTRS\\VIs\\SubPanels\\DB UI - Logon.vi\nOR \n..\\SRTRS\\SRTRS.exe\\SubPanels\\DB UI - Logon.vi"
                # "Current VI's Path\n..\\SRTRS\\VIs\\Main.vi\nOR \n..\\SRTRS\\SRTRS.exe\\Main.vi"
                # "Panel Size not Writable only Readable"
                # "Not Running YET"
                n338 = local read "Logon"() -> (w565:T21)
                n339 = local read "Update English Captions"() -> (w561:bool)
                n340 = property class="VI"(reference=w577, error in=w585) -> (error out=w584:errorcluster, "Panel"=w586:refnum<vi>)  [unwired: 1 out]
                n341 = Unbundle By Name(w565) -> ("LanguageID"=w559:string)
                n342 = To Upper Case(1:w559) -> (0:w563:string)
                n343 = Not Equal?(x=w563, y="EN") -> (x != y?=w562:bool)
                n344 = property class="Pnl"(reference=w586, error in=w584) -> (error out=w567:errorcluster, "Panes[]"=w582:refnum<vi>[], "Controls[]"=w570:refnum<vi>[])  [unwired: 1 out]
                n345 = case shown="\"Admin\"..\"Logon\"" w569 {
                  tunnel: w570 -> [_ w603]
                  tunnel: [w599 w601] -> w568
                  tunnel: w567 -> [w599 w600]
                  frame "Setup", Default {
                  }
                  frame "Admin".."Logon" {
                    # "Application Control must NOT be inside a Tab"
                    n346 = control-ref of="Application"() -> (w602:refnum<vi>)
                    n347 = call "subPanel - Write Value.vi"("Error In"=w600, "CtlRef Controls[]"=w603, "Pnl Control"=w602) -> ("Error Out"=w601:errorcluster)  [unwired: 6 in, 2 out]
                  }
                }
                n348 = Or(x=w561, y=w562) -> (x .or. y?=w560:bool)
                n349 = Index Array(array=w582, index=0) -> (element=w578:refnum<vi>)
                n350 = case shown="True" w560 {
                  tunnel: w566 -> [_ w587]
                  tunnel: w559 -> [_ w588]
                  frame False {
                  }
                  frame True {
                    n351 = case shown="Default" w587 {
                      tunnel: w587 -> [_ w598]
                      tunnel: w588 -> [_ w597]
                      frame "", "DB UI - Logon.vi" {
                        # "Skip Logon"
                      }
                      frame Default {
                        n352 = Concatenate Strings("SubPanels\\", w598) -> (w590:string)
                        n353 = local read "Current VI's path"() -> (w596:path)
                        n354 = control-ref of="MasterData\\Language"() -> (w594:refnum<vi>)
                        n355 = call "String - Create Caption Paths.vi"("LanguageID"=w597, "name or relative path"=w590, "Current VI's path"=w596, "Path in"=w594) -> ("xml Path"=w592:path, "VI Path"=w595:path)  [unwired: 6 in]
                        n356 = call "Caption Main VI.vi"("Read/Write(T) XML"=FALSE, "Read xml path"=w592, "VI path"=w595) -> ("Error Out"=w589:errorcluster)  [unwired: 8 in]
                        n357 = local write "Caption Error Out"(w589) -> ()
                      }
                    }
                  }
                }
                n358 = property class="Pane"(reference=w578, error in=w568, "HorizScrollbarVisibility"=w580, "VertScrollbarVisibility"=w580, "Origin"=T32 {"Horizontal"=0, "Vertical"=0}) -> (error out=w558:errorcluster)  [unwired: 1 out]
                n359 = invoke class="VI" method="Run VI"(reference=w577, error in=w558, "Wait until done"=FALSE ("Wait Until Done"), "Auto Dispose Ref"=FALSE ("Auto Dispose Reference")) -> (reference out=w571:refnum<vi>, error out=w572:errorcluster)  [unwired: 1 in, 3 out]
                n360 = invoke on="Invoke Node" class="SubPnl" method="Insert VI"(reference=w575, error in=w572, "VI Ref"=w571) -> (error out=w583:errorcluster)  [unwired: 1 in, 3 out]
              }
            }
            n361 = property class="SubPnl"(reference=w518) -> ("Label.Text"=w517:string)  [unwired: 1 in, 2 out]
            n362 = Concatenate Strings("[", w517, "]") -> (w516:string)
            n363 = case shown="No Error" w525 {
              tunnel: [w605 w609] -> w506
              tunnel: w516 -> [w606 w608]
              tunnel: w520 -> [w604 _]
              frame No Error {
                # "Open SubPanel OK"
                n364 = Concatenate Strings(w606, w604) -> (w605:string)
              }
              frame Error {
                # "Open SubPanel  ERROR"
                n365 = Concatenate Strings(w608, "UI Error Loading.", "\n") -> (w609:string)
              }
            }
            n366 = call "Queue - EnQueue to MessageQ.vi"("<NoD> Don't Display to UI"=TRUE, "Message"=w506) -> ()  [unwired: 9 in, 1 out]
          }
          frame "Report" {
            # "Search 7 days ahead"
            n367 = flat-sequence "Also Called in Logon" {
              frame #0 {
                w613 = ""
                w624 = 60 ("y")
                # "Initialize Report Tab"
                n368 = Get Date/Time In Seconds() -> (seconds since 1Jan1904=w627:timestamp)
                n369 = Multiply(x=7, y=24) -> (x*y=w622:i32)
                n370 = Format Date/Time String(time format string (%c)="%m") -> (date/time string=w615:string)  [unwired: 2 in]
                n371 = Format Date/Time String(time format string (%c)="%Y") -> (date/time string=w616:string)  [unwired: 2 in]
                n372 = Multiply(x=w622, y=w624) -> (x*y=w623:i32)
                n373 = property on="Selection Transaction No" class="CmbBox (strict)"("Value"=w613) -> ()  [unwired: 2 in, 2 out]
                n374 = property on="Selection Order No" class="CmbBox (strict)"("Value"=w613) -> ()  [unwired: 2 in, 2 out]
                n375 = Multiply(x=w623, y=w624) -> (x*y=w625:i32)
                n376 = Decimal String To Number(string=w616) -> (number=w617:i32)  [unwired: 2 in, 1 out]
                n377 = Decimal String To Number(string=w615) -> (number=w614:i32)  [unwired: 2 in, 1 out]
                n378 = Subtract(x=w627, y=w625) -> (x-y=w626:timestamp)
                n379 = property on="Date End" class="AbsTime (strict)"("Value"=w627) -> ()  [unwired: 2 in, 2 out]
                n380 = property on="Date Start" class="AbsTime (strict)"("Value"=w626) -> ()  [unwired: 2 in, 2 out]
                n381 = local write "FTP Year"(w617) -> ()
                n382 = local write "FTP Month"(w614) -> ()
                n383 = disable-structure shown="Disabled" {
                  frame Disabled {
                    n384 = property on="Report Execute Search" class="Bool"("DisabledEnum"=T30."Disabled and Grayed Out" ("Disabled")) -> ()  [unwired: 2 in, 2 out]
                  }
                  frame Enabled {
                  }
                }
                n385 = property on="Report Open" class="Bool"("DisabledEnum"=T30."Disabled and Grayed Out" ("Disabled")) -> ()  [unwired: 2 in, 2 out]
              }
            }
          }
        }
      }
      event "Admin (User/Equipment) Tab": Value Change {
        w629 = ""
        # "Clears When TAB is changed"
        # "Must Create Seperate Event for Child Tab"
        n386 = event-data() -> ("NewVal"=w630:enum32{"User", "Equipment"})  [unwired: 1 in, 5 out]
        n387 = local write "[Remarks] +[ShortDescription]"(w629) -> ()
        n388 = local write "[Remarks] +[ShortDescription] Debug"(w629) -> ()
        n389 = case shown="\"Equipment\"" w630 {
          frame "User", Default {
          }
          frame "Equipment" {
            n390 = property on="Tab Body" class="TabCtl (strict)"() -> ("Value"=w631:T1)  [unwired: 2 in, 2 out]
            n391 = property on="Tab Body" class="TabCtl (strict)"("Val(Sgnl)"=w631) -> ()  [unwired: 2 in, 2 out]
          }
        }
      }
      event "Master Data Tab": Value Change {
        w632 = ""
        # "Clears When TAB is changed"
        # "Must create seperate event for Child Tab"
        n392 = event-data() -> ("NewVal"=w633:enum32{"Material", "WPS", "Layout"})  [unwired: 1 in, 5 out]
        n393 = local write "[Remarks] +[ShortDescription] Debug"(w632) -> ()
        n394 = local write "[Remarks] +[ShortDescription]"(w632) -> ()
        n395 = case shown="\"Layout\"" w633 {
          frame "Material", Default {
          }
          frame "Layout" {
            n396 = property on="Tab Body" class="TabCtl (strict)"() -> ("Value"=w634:T1)  [unwired: 2 in, 2 out]
            n397 = property on="Tab Body" class="TabCtl (strict)"("Val(Sgnl)"=w634) -> ()  [unwired: 2 in, 2 out]
          }
        }
      }
      event "Close", "Debug Close": Value Change {
        n398 = event-data() -> ()  [unwired: 1 in, 6 out]
        n399 = local read "Show Debug TAB"() -> (w637:bool)
        n400 = And(x=w637, y="Debug Close") -> (x .and. y?=w635:bool)
        n401 = case shown="False" w635 {
          tunnel: [w640 w713] -> w638
          frame False {
            # "Close OR Log off"
            n402 = property on="Close" class="Bool (strict)"() -> ("BoolText.Text"=w639:string)  [unwired: 2 in, 2 out]
            n403 = case shown="\"Log off\", Default" w639 {
              tunnel: [FALSE ("T button?") w700 w710] -> w640
              frame "Log off", Default {
                n404 = First Call?() -> (First Call?: T/F=w642:bool)
                n405 = case shown="False" w642 {
                  tunnel: [w648 TRUE ("T button?")] -> w643
                  frame False {
                    # "Prompt on subsequent Log off"
                    n406 = call "Msgbox - Message Handler.vi"("Short Description (When DB Not Available)"="Log off Application.", "Description (When DB Not Available)"="All unsaved data will be lost. Do you want to proceed Logoff?", "<.?....> Message Code"="<W 001>") -> ("MHandler Error"=w649:errorcluster, "OK Out"=w648:bool)  [unwired: 6 in, 1 out]
                    n407 = local write "MHandler"(w649) -> ()
                  }
                  frame True {
                    (unwired) "1st Startup." ("string")
                    # "1st Startup, no prompt"
                  }
                }
                n408 = local write "Close"(FALSE ("Quit")) -> ()
                n409 = case shown="True" w643 {
                  frame False {
                  }
                  frame True {
                    # "Log off CONFIRMED"
                    n410 = flat-sequence {
                      tunnel: [errorcluster {"status"=FALSE, "code"=0, "source"=""} ("error constant")] -> w651
                      frame #0 {
                        w659 = string[][] [] ("Item Names")
                        w664 = ""
                        # "Reset to Initial Values"
                        n411 = local read "Plant and Furnace Name (B4 Logon)"() -> (w661:string)
                        n412 = global read "Global SRTRS.vi" "Logon Extra"() -> (w666:T25)
                        n413 = Bundle By Name(cluster=w666, "UserName"=w664) -> (w665:T25)
                        n414 = local write "Plant and Furnace Name"(w661) -> ()
                        n415 = global read "Global SRTRS.vi" "Logon"() -> (w668:T21)
                        n416 = Bundle By Name(cluster=w668, "UserID"=w664) -> (w667:T21)
                        n417 = local write "Raw Data File (Report Tab)"(path "" ("Raw Data File (Report Tab)")) -> ()
                        n418 = local write "Logon OK"(FALSE ("Logon OK")) -> ()
                        n419 = property on="Setup New Toggle" class="Bool (strict)"("Val(Sgnl)"=TRUE) -> ()  [unwired: 2 in, 2 out]
                        n420 = property on="Master Data WPS/Ref" class="CmbBox (strict)"("Val(Sgnl)"="") -> ()  [unwired: 2 in, 2 out]
                        n421 = global write "Global SRTRS.vi" "Logon Extra"(w665) -> ()
                        n422 = global write "Global SRTRS.vi" "Logon"(w667) -> ()
                        n423 = property on="Report List" class="MCListbox (strict)"("ItemNames"=w659) -> ()  [unwired: 2 in, 2 out]
                        n424 = property on="FTP File List" class="MCListbox (strict)"("ItemNames"=w659) -> ()  [unwired: 2 in, 2 out]
                      }
                    }
                    n425 = local read "DB - Logon"() -> (w653:bool)
                    n426 = local read "Lite Version"() -> (w655:bool)
                    n427 = local read "Show Debug TAB"() -> (w654:bool)
                    n428 = property on="Tab Body" class="TabCtl (strict)"() -> ("Pages"=w652:refnum<vi>[])  [unwired: 2 in, 2 out]
                    n429 = case shown="False" w653 {
                      tunnel: w654 -> [w675 w689]
                      tunnel: w655 -> [w674 _]
                      tunnel: [w673 Enum_-_Tabs."Logon" ("Tab Body")] -> w656
                      tunnel: w652 -> [w670 w687]
                      tunnel: w651 -> [w669 _]
                      frame False {
                        # "Set TAB to Report Tab \nin Lite Version"
                        n430 = for {
                          tunnel: w670 -> [w682] mode=indexing
                          tunnel: w675 -> [w681]
                          tunnel: w674 -> [w678]
                          tunnel: w669 -> [w676]
                          (unwired) "Debug" ("y")
                          n431 = property class="Page"(reference=w682, error in=w676) -> (reference out=w677:refnum<vi>, "PageLabel"=w680:string)  [unwired: 1 out]
                          n432 = case shown="\"Debug\"" w680 {
                            tunnel: w681 -> [_ w685 _]
                            tunnel: [w683 w685 TRUE] -> w679
                            tunnel: w678 -> [w684 _ _]
                            frame "Execute", "Setup", Default {
                              # "If Lite Version\nthese TAB will be hidden"
                              n433 = Not(x=w684) -> (.not. x?=w683:bool)
                            }
                            frame "Debug" {
                              # "Debug dependent of \n\"Show Debug Tab ONLY\""
                            }
                            frame "Master Data", "Report" {
                              # "These Tabs ALWAYS shown"
                            }
                          }
                          n434 = property class="Page"(reference=w677, "PageVis"=w679) -> ()  [unwired: 1 in, 2 out]
                        }
                        n435 = Select(t=Enum_-_Tabs."Report" ("Tab Body"), s=w674, f=Enum_-_Tabs."Setup" ("Tab Body")) -> (s? t:f=w673:T42)
                      }
                      frame True {
                        # "Use DB to Logon"
                        n436 = for {
                          tunnel: w687 -> [w694] mode=indexing
                          tunnel: w689 -> [w693]
                          (unwired) "Debug" ("y")
                          n437 = property class="Page"(reference=w694) -> (reference out=w690:refnum<vi>, "PageLabel"=w692:string)  [unwired: 1 in, 1 out]
                          n438 = case shown="\"Setup\", Default" w692 {
                            tunnel: w693 -> [_ w696 _]
                            tunnel: [FALSE ("Show Debug Tab") w696 TRUE] -> w691
                            frame "Setup", Default {
                              # "All\nthese TAB will be hidden"
                            }
                            frame "Debug" {
                              # "Show Debug?"
                            }
                            frame "Logon" {
                              # "These Tabs ALWAYS shown"
                            }
                          }
                          n439 = property class="Page"(reference=w690, "PageVis"=w691) -> ()  [unwired: 1 in, 2 out]
                        }
                      }
                    }
                    n440 = property on="Tab Body" class="TabCtl (strict)"("Val(Sgnl)"=w656) -> ()  [unwired: 2 in, 2 out]
                  }
                }
              }
              frame "Close" {
                n441 = call "Msgbox - Message Handler.vi"("Short Description (When DB Not Available)"="Close Application", "Description (When DB Not Available)"="Confirm close Application?", "<.?....> Message Code"="<W 104>") -> ("MHandler Error"=w702:errorcluster, "OK Out"=w700:bool)  [unwired: 6 in, 1 out]
                n442 = local write "MHandler"(w702) -> ()
                n443 = local write "Quit Flag"(w700) -> ()
                n444 = flat-sequence {
                  tunnel: [w706] -> w704
                  tunnel: "Close" -> [w706]
                  tunnel: w704 -> [_]
                  frame #0 {
                    n445 = Wait (ms)(milliseconds to wait=u32 100) -> ()  [unwired: 1 out]
                  }
                  frame #1 {
                    n446 = local write "Close"(FALSE ("Quit")) -> ()
                  }
                }
                n447 = case shown="True" w700 {
                  frame False {
                  }
                  frame True {
                    n448 = property on="Stop Log off Event Structure" class="Bool (strict)"("Val(Sgnl)"=TRUE ("Value (Signaling)")) -> ()  [unwired: 2 in, 2 out]
                  }
                }
              }
              frame "Close Now" {
